vi "GetAlarms.vi"(0 "AI in":refnum<class "AI.lvclass">, 11 "error in (no error)":errorcluster) -> (4 "AI out":refnum<class "AI.lvclass">, 6 "Alarm":bool, 8 "Warning":bool, 15 "error out":errorcluster)   [LabVIEW 2019, in "AI.lvclass"]
uses:
  AI.lvclass
  AI.lvclass/AI.ctl
  AnalogComparator_class/AnalogComparator.lvclass
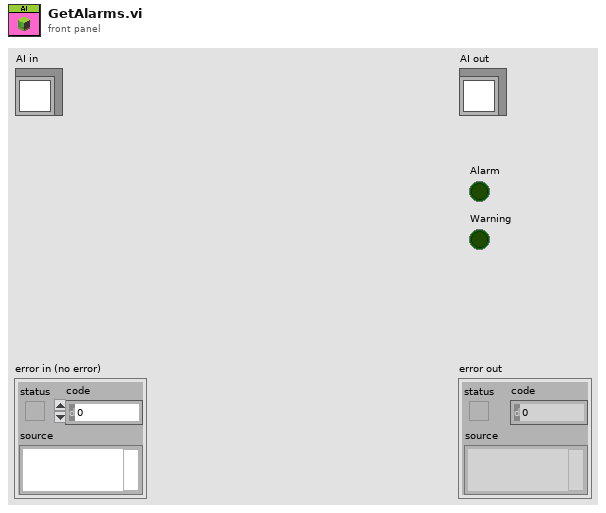
[diagram p1: front panel]
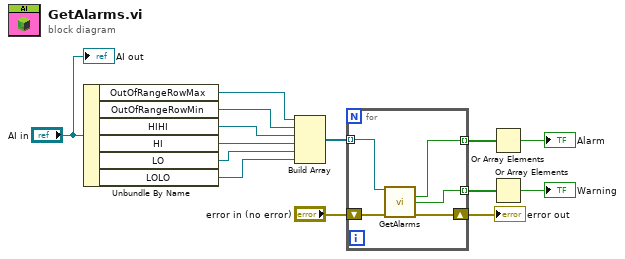
[diagram p0: block diagram]
diagram:
  n1 = Unbundle By Name("AI in") -> ("OutOfRangeRowMax"=w13:refnum<class "AnalogComparator.lvclass">, "OutOfRangeRowMin"=w12:refnum<class "AnalogComparator.lvclass">, "HIHI"=w11:refnum<class "AnalogComparator.lvclass">, "HI"=w10:refnum<class "AnalogComparator.lvclass">, "LO"=w9:refnum<class "AnalogComparator.lvclass">, "LOLO"=w8:refnum<class "AnalogComparator.lvclass">)
  n2 = Build Array(w13, w12, w11, w10, w9, w8) -> (w7:refnum<class "AnalogComparator.lvclass">[])
  n3 = for {
    tunnel: w7 -> [w19] mode=indexing
    shift-right: [w17] -> w5
    shift-left: "error in (no error)" -> [w18]
    tunnel: [w16] -> w4 mode=indexing
    tunnel: [w15] -> w3 mode=indexing
    n4 = call-dynamic "GetAlarms.vi"("AnalogComparator in"=w19, "error in (no error)"=w18) -> ("Alarm"=w16:bool, "Warning"=w15:bool, "error out"=w17:errorcluster)  [unwired: 10 in, 1 out]
  }
  "error out" <- w5
  n5 = Or Array Elements(Boolean array=w4) -> (logical OR=→"Alarm":bool)
  n6 = Or Array Elements(Boolean array=w3) -> (logical OR=→"Warning":bool)
  "AI out" <- "AI in"
